vi "Measure_Osc_Current.vi"(8 "error in":errorcluster, 10 "KeyState$":string) -> (0 "error out":errorcluster, 2 "Osc Current":dbl)   [LabVIEW 2020]
panel:
  in  "RD$":string
  # "A2B2C1D0F17H0I1M2S0T1E"
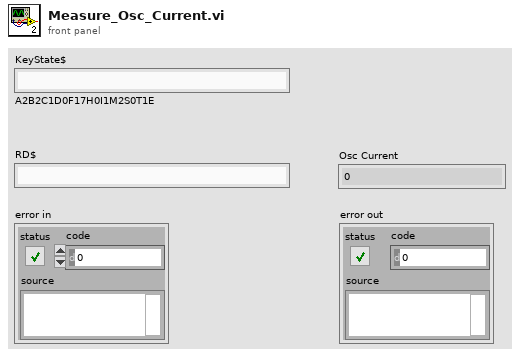
[diagram p1: front panel]
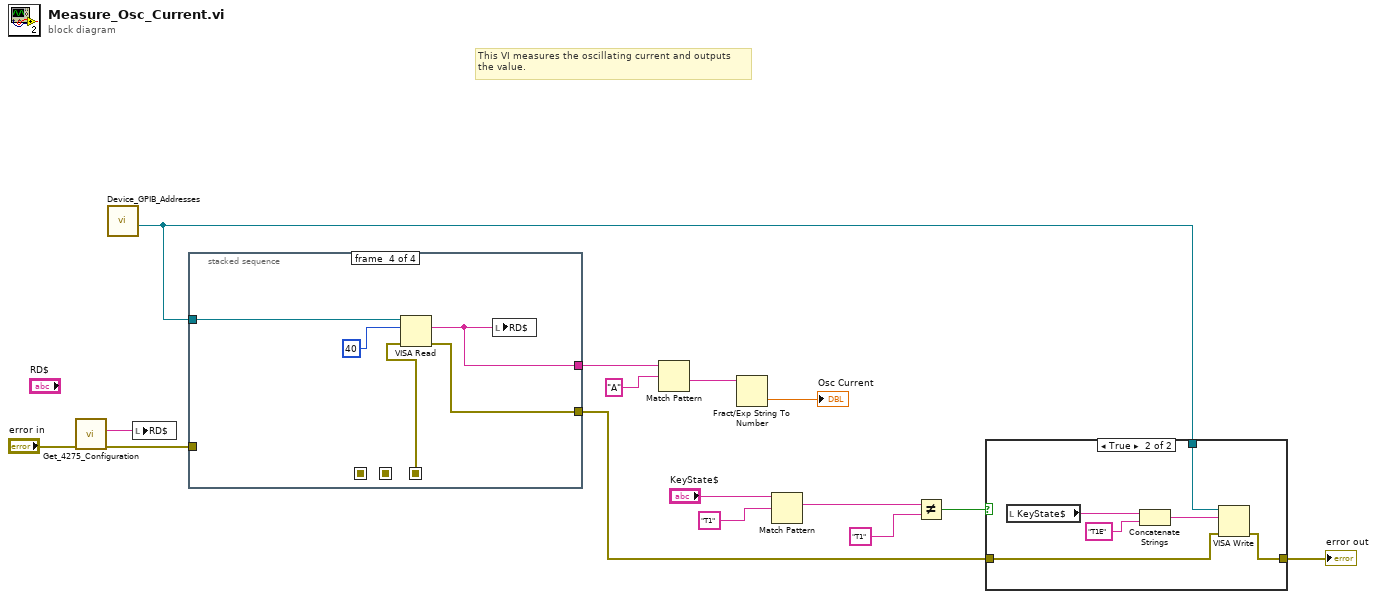
[diagram p0: block diagram]
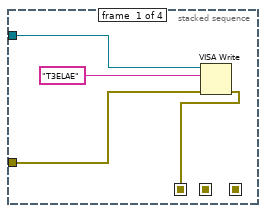
[diagram p3: hidden frame]
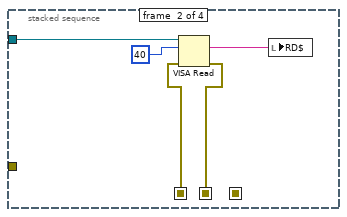
[diagram p4: hidden frame]
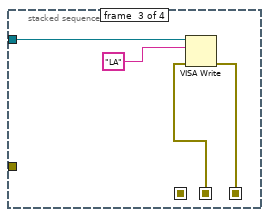
[diagram p5: hidden frame]
diagram:
  # "This VI measures the oscillating current and outputs\nthe value."
  n1 = call "Get_4275_Configuration.vi"("error in"="error in") -> ("error out"=w14:errorcluster, "Keystate"=w15:string)  [unwired: 9 in]
  n2 = call "Device_GPIB_Addresses.vi"() -> ("HP 4275A Address"=w1:refnum<visa-resource-name>)  [unwired: 9 in, 2 out]
  n3 = local write "RD$"(w15) -> ()
  n4 = stacked-sequence {
    seq-local: [w16 _ _ _] -> [_ w21 _ _]
    seq-local: [_ w20 _ _] -> [_ _ w26 _]
    seq-local: [_ _ w25 _] -> [_ _ _ w30]
    tunnel: w14 -> [w17 _ _ _]
    tunnel: [_ _ _ w33] -> w11
    tunnel: [_ _ _ w29] -> w3
    tunnel: w1 -> [w19 w24 w28 w32]
    frame #0 {
      n5 = VISA Write(VISA resource name=w19, write buffer="T3ELAE" ("data"), error in (no error)=w17) -> (error out=w16:errorcluster)  [unwired: 2 out]
    }
    frame #1 {
      n6 = VISA Read(VISA resource name=w24, byte count=40, error in (no error)=w21) -> (read buffer=w22:string, error out=w20:errorcluster)  [unwired: 2 out]
      n7 = local write "RD$"(w22) -> ()
    }
    frame #2 {
      n8 = VISA Write(VISA resource name=w28, write buffer="LA" ("data"), error in (no error)=w26) -> (error out=w25:errorcluster)  [unwired: 2 out]
    }
    frame #3 {
      n9 = VISA Read(VISA resource name=w32, byte count=40, error in (no error)=w30) -> (read buffer=w33:string, error out=w29:errorcluster)  [unwired: 2 out]
      n10 = local write "RD$"(w33) -> ()
    }
  }
  n11 = Match Pattern(string=w11, regular expression="A") -> (after substring=w10:string)  [unwired: 1 in, 3 out]
  n12 = Fract/Exp String To Number(string=w10) -> (number=→"Osc Current":dbl)  [unwired: 3 in, 1 out]
  n13 = Match Pattern(string="KeyState$", regular expression="T1") -> (match substring=w6:string)  [unwired: 1 in, 3 out]
  n14 = Not Equal?(x=w6, y="T1") -> (x != y?=w4:bool)
  n15 = case shown="True" w4 {
    tunnel: w3 -> [w34 w36]
    tunnel: [w34 w35] -> w2
    tunnel: w1 -> [_ w38]
    frame False {
    }
    frame True {
      n16 = local read "KeyState$"() -> (w40:string)
      n17 = Concatenate Strings(w40, "T1E" ("string")) -> (w37:string)
      n18 = VISA Write(VISA resource name=w38, write buffer=w37, error in (no error)=w36) -> (error out=w35:errorcluster)  [unwired: 2 out]
    }
  }
  "error out" <- w2
